vi "Focus_Dialog.vi"(11 "System Data":T1={"System"={"Active"=FALSE, "Exit"=FALSE, "Command wait"="", "Status_Time"=0, "Time_GPS"=0}, "Stepper Motor"={"Connection Reference"="", "Valid Connection"=FALSE, "Speed"=15}, "Camera Data"={"Image path"=path "", "Filenames"=[], "Filenames queue"=[]}, "Core"={"Close Panel on Exit?"=FALSE, "Current VI Reference"=refnum}} {"Stepper Motor"."Speed" scale=0.0..30.0}) -> (3 "System Data out":T1={"System"={"Active"=FALSE, "Exit"=FALSE, "Command wait"="", "Status_Time"=0, "Time_GPS"=0}, "Stepper Motor"={"Connection Reference"="", "Valid Connection"=FALSE, "Speed"=15}, "Camera Data"={"Image path"=path "", "Filenames"=[], "Filenames queue"=[]}, "Core"={"Close Panel on Exit?"=FALSE, "Current VI Reference"=refnum}} {"Stepper Motor"."Speed" scale=0.0..30.0})   [LabVIEW 2019]
uses:
  System Data.ctl
  Stepper Data.ctl
  Camera Data.ctl
panel:
  in  "Right":bool
  in  "Left":bool
  out "Pict Ring":dbl(ring)
  in  "Speed":i32(slide)=15 scale=0.0..20.0
  in  "OK":bool
  # "Lens Focus"
  # "Hint: use Left or Right arrow key to adjust focus"
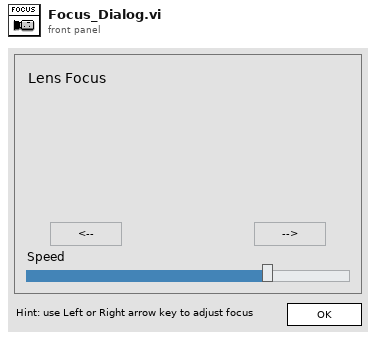
[diagram p1: front panel]
types:
  T1 = typedef "System Data.ctl" = cluster{"System":cluster{"Active":bool, "Exit":bool, "Command wait":string, "Status_Time":i32, "Time_GPS":i32}, "Stepper Motor":T2, "Camera Data":T3, "Core":cluster{"Close Panel on Exit?":bool, "Current VI Reference":refnum<vi>}}
  T2 = typedef "Stepper Data.ctl" = cluster{"Connection Reference":refnum<visa-resource-name>, "Valid Connection":bool, "Speed":i32}
  T3 = typedef "Camera Data.ctl" = cluster{"Image path":path, "Filenames":string[], "Filenames queue":string[]}
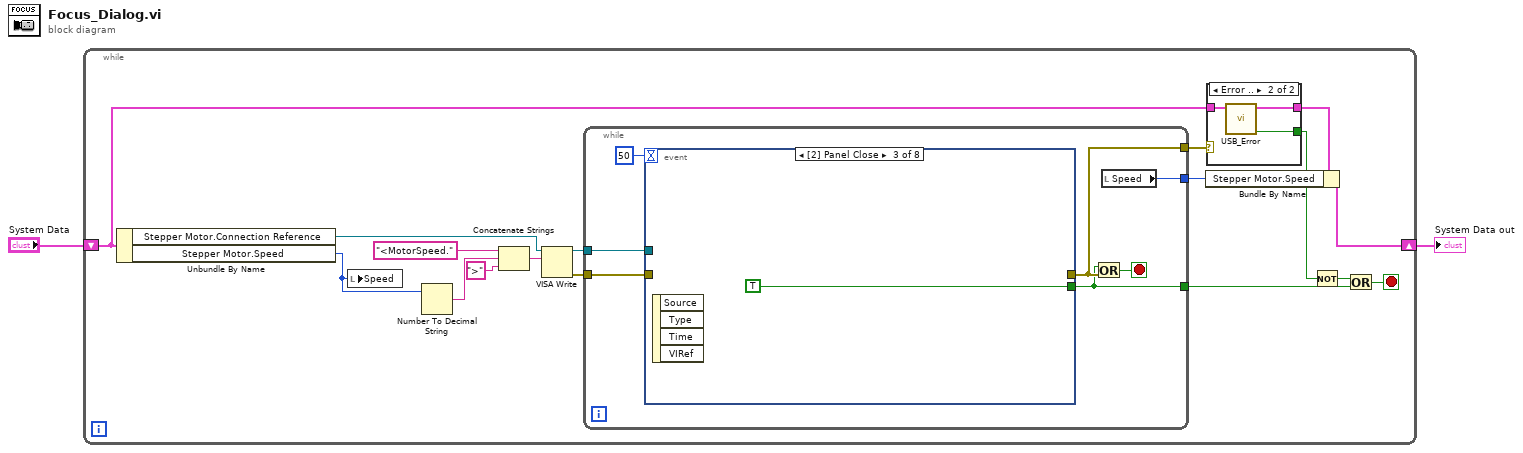
[diagram p0: block diagram]
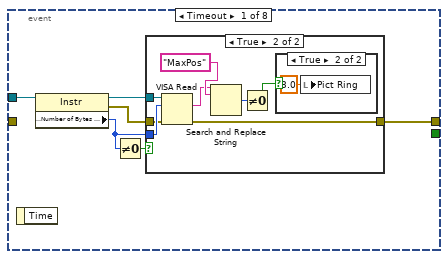
[diagram p2: hidden frame]
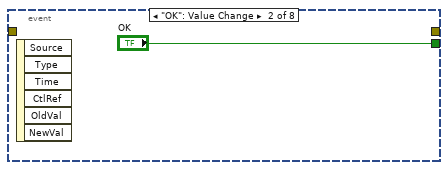
[diagram p5: hidden frame]
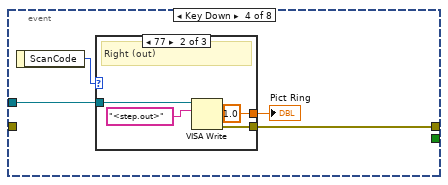
[diagram p6: hidden frame]
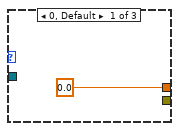
[diagram p7: hidden frame]
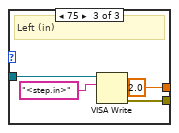
[diagram p8: hidden frame]
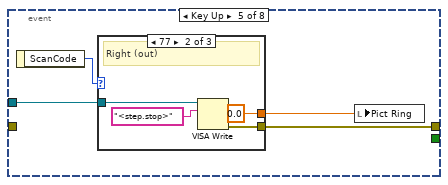
[diagram p9: hidden frame]
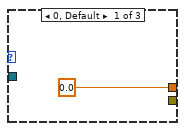
[diagram p10: hidden frame]
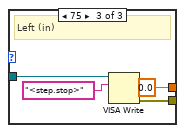
[diagram p11: hidden frame]
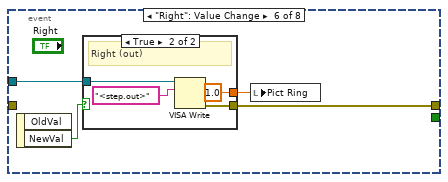
[diagram p12: hidden frame]
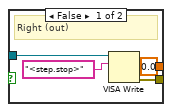
[diagram p13: hidden frame]
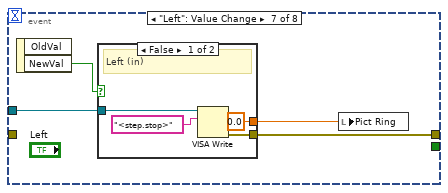
[diagram p14: hidden frame]
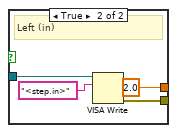
[diagram p15: hidden frame]
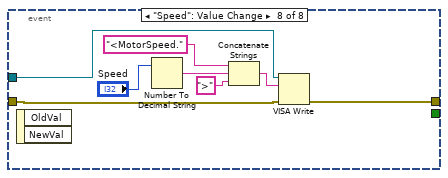
[diagram p16: hidden frame]
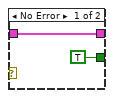
[diagram p17: hidden frame]
diagram:
  n1 = while {
    shift-right: [w3] -> w2
    shift-left: "System Data" -> [w16]
    stop <- w15 stop-if-true
    n2 = Unbundle By Name(w16) -> ("Stepper Motor.Connection Reference"=w13:refnum<visa-resource-name>, "Stepper Motor.Speed"=w8:i32)
    n3 = local write "Speed"(w8) -> ()
    n4 = Number To Decimal String(number=w8) -> (decimal integer string=w11:string)  [unwired: 1 in]
    n5 = Concatenate Strings("<MotorSpeed." ("write buffer"), w11, ">" ("string")) -> (w7:string)
    n6 = VISA Write(VISA resource name=w13, write buffer=w7) -> (VISA resource name out=w12:refnum<visa-resource-name>, error out=w6:errorcluster)  [unwired: 1 in, 1 out]
    n7 = while {
      tunnel: w12 -> [w22]
      tunnel: [w24] -> w19
      tunnel: [w23] -> w14
      tunnel: w6 -> [w21]
      tunnel: [w20] -> w5
      stop <- w25 stop-if-true
      n8 = event shown="[2] Panel Close" {
        selector: _ -> [_ _ _ _ _ _ _ _]
        dyn-events: _ -> [_ _ _ _ _ _ _ _]
        timeout: 50 -> [_ _ _ _ _ _ _ _]
        tunnel: [_ "OK" TRUE ("OK") _ _ _ _ _] -> w23
        tunnel: w22 -> [w29 _ _ w47 w60 w74 w86 w102]
        tunnel: [w27 _ _ w45 w58 w72 w84 w97] -> w24
        tunnel: w21 -> [_ _ _ _ _ _ _ w96]
        event Timeout {
          n9 = event-data() -> ()  [unwired: 1 in, 1 out]
          n10 = property class="Instr"(reference=w29) -> (reference out=w32:refnum<visa-resource-name>, error out=w28:errorcluster, "Serial Settings:Number of Bytes at Serial Port"=w31:u32)  [unwired: 1 in]
          n11 = Not Equal To 0?(x=w31) -> (x != 0?=w30:bool)
          n12 = case shown="True" w30 {
            tunnel: w32 -> [_ w41]
            tunnel: w31 -> [_ w40]
            tunnel: w28 -> [w33 w39]
            tunnel: [w33 w38] -> w27
            frame False {
            }
            frame True {
              n13 = VISA Read(VISA resource name=w41, byte count=w40, error in (no error)=w39) -> (read buffer=w35:string, error out=w38:errorcluster)  [unwired: 2 out]
              n14 = Search and Replace String(input string=w35, search string="MaxPos") -> (number of replacements=w37:i32)  [unwired: 6 in, 3 out]
              n15 = Not Equal To 0?(x=w37) -> (x != 0?=w34:bool)
              n16 = case shown="True" w34 {
                frame False {
                }
                frame True {
                  n17 = local write "Pict Ring"(3.0 ("Pict Ring")) -> ()
                }
              }
            }
          }
        }
        event "OK": Value Change {
          n18 = event-data() -> ()  [unwired: 1 in, 6 out]
        }
        event Panel Close {
          n19 = event-data() -> ()  [unwired: 1 in, 4 out]
        }
        event Key Down {
          n20 = event-data() -> ("ScanCode"=w48:i16)  [unwired: 1 in]
          n21 = case shown="77" w48 {
            tunnel: w47 -> [_ w52 w56]
            tunnel: [0.0 ("Pict Ring") 1.0 ("Pict Ring") 2.0 ("Pict Ring")] -> w46
            tunnel: [_ w50 w54] -> w45
            frame 0, Default {
            }
            frame 77 {
              # "Right (out)"
              n22 = VISA Write(VISA resource name=w52, write buffer="<step.out>") -> (error out=w50:errorcluster)  [unwired: 1 in, 2 out]
            }
            frame 75 {
              # "Left (in)"
              n23 = VISA Write(VISA resource name=w56, write buffer="<step.in>") -> (error out=w54:errorcluster)  [unwired: 1 in, 2 out]
            }
          }
          "Pict Ring" <- w46
        }
        event Key Up {
          n24 = event-data() -> ("ScanCode"=w61:i16)  [unwired: 1 in]
          n25 = case shown="77" w61 {
            tunnel: w60 -> [_ w66 w69]
            tunnel: [0.0 ("Pict Ring") 0.0 ("Pict Ring") 0.0 ("Pict Ring")] -> w59
            tunnel: [_ w63 w67] -> w58
            frame 0, Default {
            }
            frame 77 {
              # "Right (out)"
              n26 = VISA Write(VISA resource name=w66, write buffer="<step.stop>") -> (error out=w63:errorcluster)  [unwired: 1 in, 2 out]
            }
            frame 75 {
              # "Left (in)"
              n27 = VISA Write(VISA resource name=w69, write buffer="<step.stop>") -> (error out=w67:errorcluster)  [unwired: 1 in, 2 out]
            }
          }
          n28 = local write "Pict Ring"(w59) -> ()
        }
        event "Right": Value Change {
          n29 = event-data() -> ("NewVal"=w71:bool)  [unwired: 1 in, 1 out]
          n30 = case shown="True" w71 {
            tunnel: w74 -> [w78 w81]
            tunnel: [0.0 ("Pict Ring") 1.0 ("Pict Ring")] -> w73
            tunnel: [w75 w79] -> w72
            frame False {
              # "Right (out)"
              n31 = VISA Write(VISA resource name=w78, write buffer="<step.stop>") -> (error out=w75:errorcluster)  [unwired: 1 in, 2 out]
            }
            frame True {
              # "Right (out)"
              n32 = VISA Write(VISA resource name=w81, write buffer="<step.out>") -> (error out=w79:errorcluster)  [unwired: 1 in, 2 out]
            }
          }
          n33 = local write "Pict Ring"(w73) -> ()
        }
        event "Left": Value Change {
          n34 = event-data() -> ("NewVal"=w83:bool)  [unwired: 1 in, 1 out]
          n35 = case shown="False" w83 {
            tunnel: w86 -> [w90 w93]
            tunnel: [0.0 ("Pict Ring") 2.0 ("Pict Ring")] -> w85
            tunnel: [w87 w91] -> w84
            frame False {
              # "Left (in)"
              n36 = VISA Write(VISA resource name=w90, write buffer="<step.stop>") -> (error out=w87:errorcluster)  [unwired: 1 in, 2 out]
            }
            frame True {
              # "Left (in)"
              n37 = VISA Write(VISA resource name=w93, write buffer="<step.in>") -> (error out=w91:errorcluster)  [unwired: 1 in, 2 out]
            }
          }
          n38 = local write "Pict Ring"(w85) -> ()
        }
        event "Speed": Value Change {
          n39 = event-data() -> ()  [unwired: 1 in, 2 out]
          n40 = Number To Decimal String(number="Speed") -> (decimal integer string=w98:string)  [unwired: 1 in]
          n41 = Concatenate Strings("<MotorSpeed." ("write buffer"), w98, ">" ("string")) -> (w100:string)
          n42 = VISA Write(VISA resource name=w102, write buffer=w100, error in (no error)=w96) -> (error out=w97:errorcluster)  [unwired: 2 out]
        }
      }
      n43 = Or(x=w23, y=w24) -> (x .or. y?=w25:bool)
      n44 = local read "Speed"() -> (w20:i32)
    }
    n45 = case shown="Error .." w19 {
      tunnel: w16 -> [w103 w107]
      tunnel: [TRUE ("Connection") w106] -> w17
      tunnel: [w103 w105] -> w4
      frame No Error {
      }
      frame Error {
        n46 = call "USB_Error.vi"("System Data"=w107) -> ("Connection"=w106:bool, "System Data out"=w105:T1)  [unwired: 9 in]
      }
    }
    n47 = Bundle By Name(cluster=w4, "Stepper Motor.Speed"=w5) -> (w3:T1)
    n48 = Not(x=w17) -> (.not. x?=w18:bool)
    n49 = Or(x=w18, y=w14) -> (x .or. y?=w15:bool)
  }
  "System Data out" <- w2
